vi "write_params.vi"(8 "error in (no error)":errorcluster, 10 "params":T1={"estimators"=[], "weights"={"weights_type"="None", "weights_list"=[]}, "n_jobs"=1.0, "verbose"=FALSE}, 11 "VotingRegressor in":refnum<class "VotingRegressor.lvclass">) -> (0 "error out":errorcluster, 3 "VotingRegressor out":refnum<class "VotingRegressor.lvclass">)   [LabVIEW 2020, in "VotingRegressor.lvclass"]
uses:
  VotingRegressor.lvclass
  Controls/voting_regressor_params.ctl
  VotingRegressor.lvclass/VotingRegressor.ctl
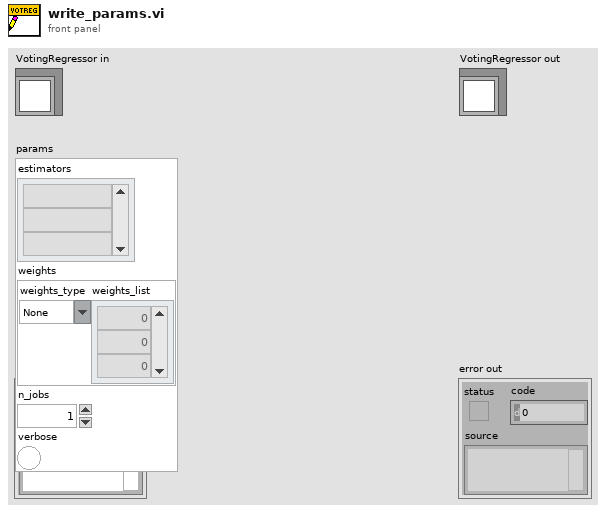
[diagram p1: front panel]
types:
  T1 = typedef "voting_regressor_params.ctl" = cluster{"estimators":string[], "weights":cluster{"weights_type":string, "weights_list":dbl[]}, "n_jobs":dbl, "verbose":bool}
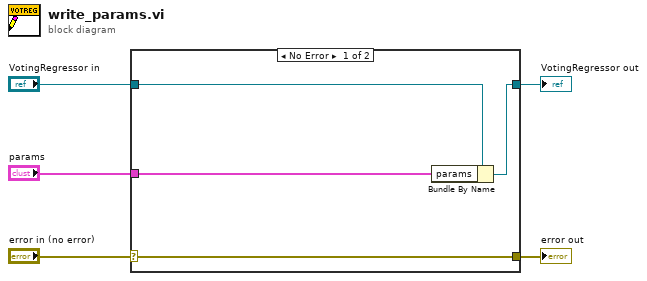
[diagram p0: block diagram]
diagram:
  n1 = case shown="No Error" "error in (no error)" {
    selector: "error in (no error)" -> [w9 w10]
    tunnel: [w9 w10] -> w4
    tunnel: [w7 w11] -> w2
    tunnel: "VotingRegressor in" -> [w8 w11]
    tunnel: "params" -> [w6 _]
    frame No Error {
      n2 = Bundle By Name(cluster=w8, "params"=w6) -> (w7:refnum<class "VotingRegressor.lvclass">)
    }
    frame Error {
    }
  }
  "error out" <- w4
  "VotingRegressor out" <- w2
